vi "INIT.vi"(8 "error in (no error)":errorcluster, 11 "Nestle_Actor in":refnum<class "Nestle_Actor.lvclass">) -> (0 "error out":errorcluster, 3 "Nestle_Actor out":refnum<class "Nestle_Actor.lvclass">)   [LabVIEW 2019, in "Nestle_Actor.lvlib" / "Nestle_Actor.lvclass"]
uses:
  Nestle_Actor.lvclass
  Nestle_Actor.lvclass/Nestle_Actor.ctl
  <vilib>/Utility/config.llb/Read Key (Double).vi
  <vilib>/Utility/config.llb/Read Key (String).vi
  <vilib>/Utility/config.llb/NI_LVConfig.lvlib
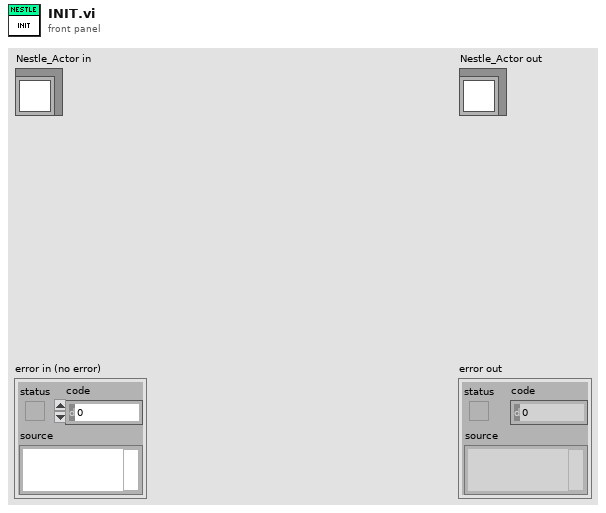
[diagram p1: front panel]
types:
  T1 = typedef "NI_LVConfig.lvlib/Config Data RefNum.ctl" = refnum<k1>
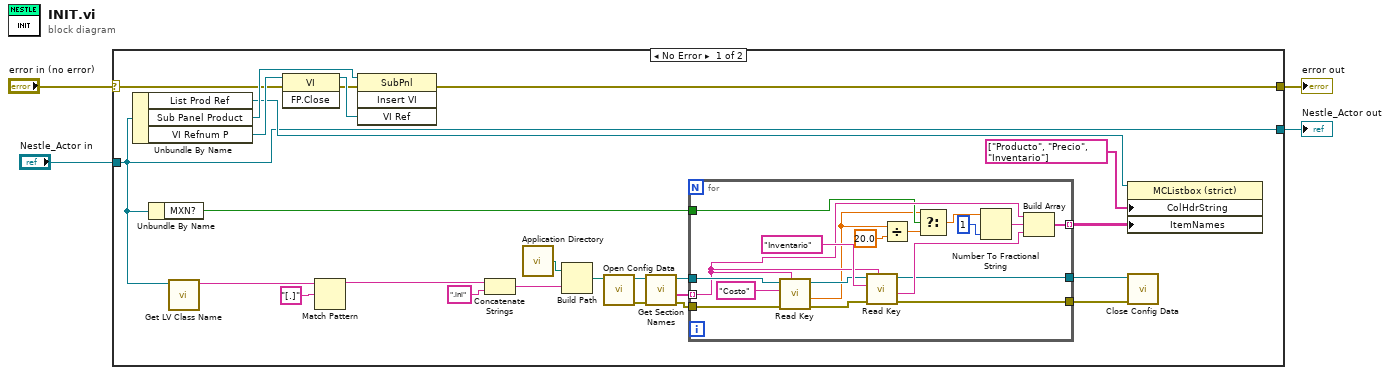
[diagram p0: block diagram]
diagram:
  n1 = case shown="No Error" "error in (no error)" {
    selector: "error in (no error)" -> [w25 w49]
    tunnel: [w24 w49] -> w3
    tunnel: [w15 w48] -> w1
    tunnel: "Nestle_Actor in" -> [w15 w48]
    frame No Error {
      n2 = Unbundle By Name(w15) -> ("List Prod Ref"=w23:refnum<vi>, "Sub Panel Product"=w28:refnum<vi>, "VI Refnum P"=w29:refnum<vi>)
      n3 = Unbundle By Name(w15) -> ("MXN?"=w5:bool)
      n4 = call <vilib>:"Get LV Class Name.vi"("object"=w15) -> ("class name"=w17:string)  [unwired: 9 in, 1 out]
      n5 = invoke class="VI" method="FP.Close"(reference=w29, error in=w25) -> (reference out=w27:refnum<vi>, error out=w26:errorcluster)  [unwired: 1 in, 1 out]
      n6 = Match Pattern(string=w17, regular expression="[.]") -> (before substring=w16:string)  [unwired: 1 in, 3 out]
      n7 = invoke class="SubPnl" method="Insert VI"(reference=w28, error in=w26, "VI Ref"=w27) -> (error out=w24:errorcluster)  [unwired: 1 in, 3 out]
      n8 = Concatenate Strings(w16, ".ini" ("string")) -> (w21:string)
      n9 = call <vilib>:"Application Directory.vi"() -> ("Application Directory"=w22:path)
      n10 = Build Path(base path=w22, name or relative path=w21) -> (appended path=w19:path)
      n11 = call <vilib>:"Open Config Data.vi"("configuration file path"=w19) -> ("error out"=w11:errorcluster, "refnum"=w13:T1)  [unwired: 8 in, 1 out]
      n12 = call <vilib>:"Get Section Names.vi"("error in (no error)"=w11, "refnum"=w13) -> ("error out"=w10:errorcluster, "section names"=w9:string[], "refnum out"=w12:T1)  [unwired: 7 in]
      n13 = for {
        tunnel: w12 -> [w44]
        tunnel: w10 -> [w45]
        tunnel: w9 -> [w41] mode=indexing
        tunnel: [w39] -> w8 mode=indexing
        tunnel: [w38] -> w7
        tunnel: [w37] -> w6
        tunnel: w5 -> [w34]
        n14 = call-poly <vilib>:"Read Key.vi"("section"=w41, "error in (no error)"=w45, "key"="Costo", "refnum"=w44) -> ("error out"=w42:errorcluster, "value"=w31:dbl, "refnum out"=w43:T1)  [unwired: 4 in, 1 out]
        n15 = call-poly <vilib>:"Read Key.vi"("section"=w41, "error in (no error)"=w42, "key"="Inventario", "refnum"=w43) -> ("error out"=w38:errorcluster, "value"=w40:string, "refnum out"=w37:T1)  [unwired: 4 in, 1 out]
        n16 = Divide(x=w31, y=20.0) -> (x/y=w32:dbl)
        n17 = Select(t=w31, s=w34, f=w32) -> (s? t:f=w33:dbl)
        n18 = Number To Fractional String(number=w33, precision (6)=i16 1) -> (F-format string=w35:string)  [unwired: 2 in]
        n19 = Build Array(w41, w35, w40) -> (w39:string[])
      }
      n20 = property class="MCListbox (strict)"(reference=w23, "ColHdrString"=string[] ["Producto", "Precio", "Inventario"] ("Column Header Strings[]"), "ItemNames"=w8) -> ()  [unwired: 1 in, 2 out]
      n21 = call <vilib>:"Close Config Data.vi"("error in (no error)"=w7, "refnum"=w6) -> ()  [unwired: 8 in, 2 out]
    }
    frame Error {
    }
  }
  "error out" <- w3
  "Nestle_Actor out" <- w1
